vi "Lambda Genesys Device Properties.vi"() -> ()   [LabVIEW 2014, in "Lambda Genesys Custom Device.lvlib"]
uses:
  Lambda Genesys Custom Device.lvlib
panel:
  in  "Baud Rate":string="Baud Rate"
  in  "Address":string="Address"
  in  "Resource":string="VISA Resource"
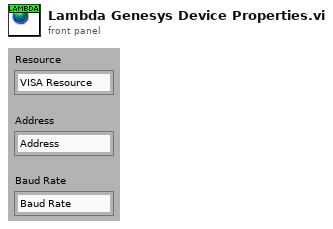
[diagram p1: front panel]
diagram:
